vi "Hypotenuse.vi"(1 "y":dbl, 2 "x":dbl) -> (0 "r":dbl)   [LabVIEW 2015, in "Navigation2017.lvlib" / "Navigation2017-util.lvlib"]
uses:
  Navigation2017-util.lvlib
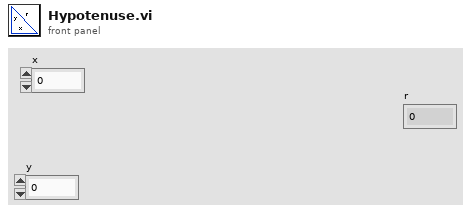
[diagram p1: front panel]
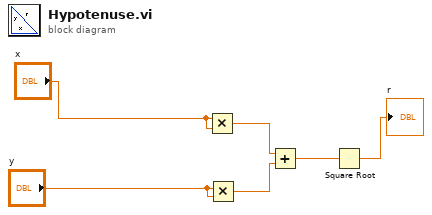
[diagram p0: block diagram]
diagram:
  n1 = Multiply(x="x", y="x") -> (x*y=w4:dbl)
  n2 = Multiply(x="y", y="y") -> (x*y=w3:dbl)
  n3 = Add(x=w4, y=w3) -> (x+y=w2:dbl)
  n4 = Square Root(x=w2) -> (sqrt(x)=→"r":dbl)
